vi "ni579x Validate EEPROM Range.vi"(0 "Register Bus":refnum<class "ni579x Register Bus v1 Host.lvclass">=refnum, 1 "scope":string, 5 "start address":u32 format="%x", 7 "size":u32, 11 "Error In":errorcluster) -> (4 "Register Bus (out)":refnum<class "ni579x Register Bus v1 Host.lvclass">, 6 "coerced start address":u32 format="%x", 8 "coerced size":u32, 15 "Error Out":errorcluster)   [LabVIEW 2013]
uses:
  <instrlib>/ni579x/Register Bus/v1/Host/ni579x Register Bus v1 Host.lvclass
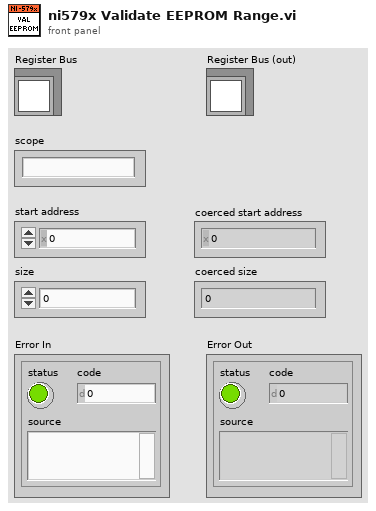
[diagram p1: front panel]
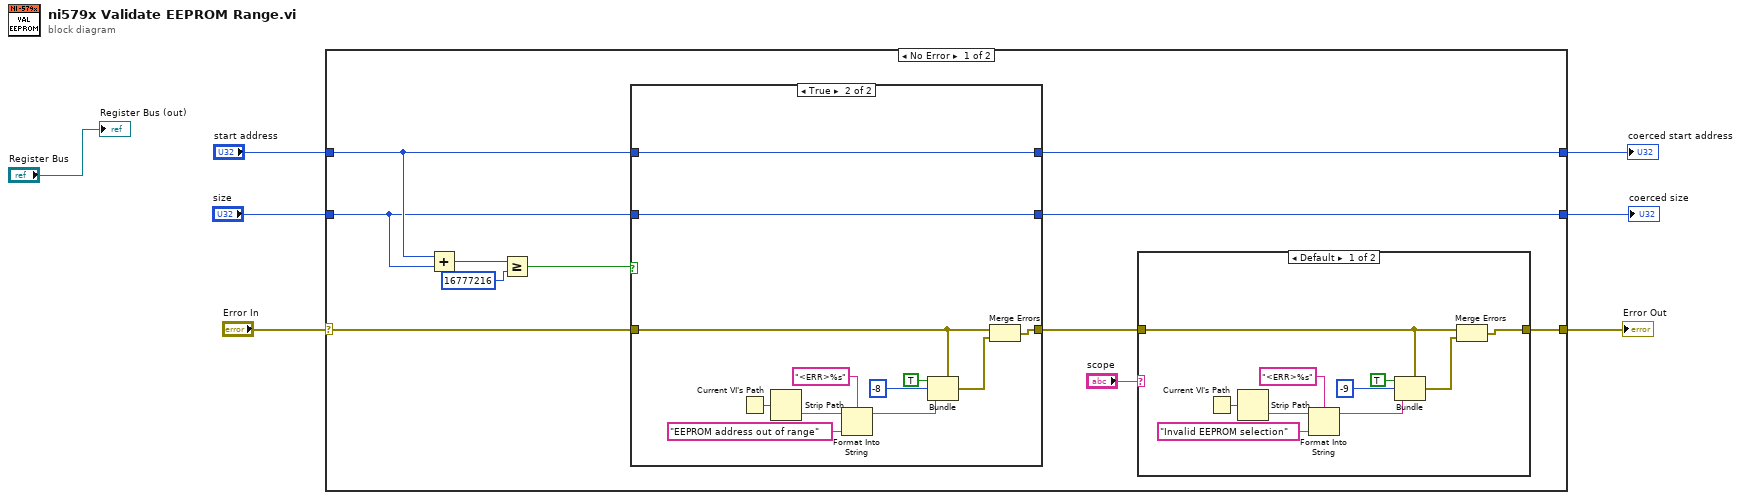
[diagram p0: block diagram]
diagram:
  n1 = case shown="No Error" "Error In" {
    selector: "Error In" -> [w18 w47]
    tunnel: [w13 w47] -> w6
    tunnel: [w17 w45] -> w3
    tunnel: [w16 w46] -> w4
    tunnel: "start address" -> [w9 w46]
    tunnel: "size" -> [w8 w45]
    frame No Error {
      n2 = Add(x=w9, y=w8) -> (x+y=w12:u32)
      n3 = Greater Or Equal?(x=w12, y=u32 16777216) -> (x >= y?=w10:bool)
      n4 = case shown="True" w10 {
        tunnel: w8 -> [w31 w37]
        tunnel: [w31 w37] -> w17
        tunnel: w18 -> [w32 w40]
        tunnel: [w32 w38] -> w14
        tunnel: [w30 w33] -> w16
        tunnel: w9 -> [w30 w33]
        frame False {
        }
        frame True {
          n5 = Current VI's Path() -> (path=w43:path)
          n6 = Strip Path(path=w43) -> (name=w42:string)  [unwired: 1 out]
          n7 = Format Into String(format string="<ERR>%s", initial string=w42, "EEPROM address out of range" ("input 1")) -> (resulting string=w41:string)  [unwired: 1 in, 1 out]
          n8 = Bundle(cluster=w40, "status"=TRUE, "code"=-8, "source"=w41) -> (w39:errorcluster)
          n9 = Merge Errors(w40, w39) -> (w38:errorcluster)
        }
      }
      n10 = case shown="Default" "scope" {
        tunnel: w14 -> [w21 w29]
        tunnel: [w19 w29] -> w13
        frame Default {
          n11 = Current VI's Path() -> (path=w23:path)
          n12 = Strip Path(path=w23) -> (name=w24:string)  [unwired: 1 out]
          n13 = Format Into String(format string="<ERR>%s", initial string=w24, "Invalid EEPROM selection" ("input 1")) -> (resulting string=w25:string)  [unwired: 1 in, 1 out]
          n14 = Bundle(cluster=w21, "status"=TRUE, "code"=-9, "source"=w25) -> (w20:errorcluster)
          n15 = Merge Errors(w21, w20) -> (w19:errorcluster)
        }
        frame "characterization data eeprom" {
        }
      }
    }
    frame Error {
    }
  }
  "Error Out" <- w6
  "coerced start address" <- w4
  "coerced size" <- w3
  "Register Bus (out)" <- "Register Bus"
